vi "Ctor.vi"(8 "error in (no error)":errorcluster) -> (0 "error out":errorcluster, 3 "nmea out":refnum<class "nmea.lvclass">)   [LabVIEW 2012, in "nmea.lvlib" / "nmea.lvclass"]
uses:
  nmea.lvclass
  Ref Data.ctl
  <vilib>/Utility/miscctls.llb/LVDateTimeRec.ctl
  Satellite.ctl
  Fix Type.ctl
  DOP.ctl
  Fix Mode.ctl
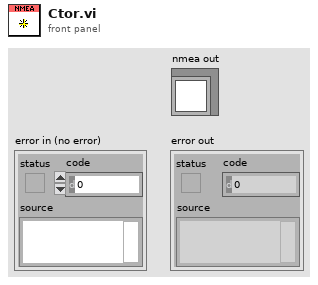
[diagram p1: front panel]
types:
  T1 = typedef "nmea.lvlib/nmea.lvclass/Ref Data.ctl" = cluster{"Latitude":dbl, "Longitude":dbl, "Time":T2, "Status":string, "Speed":dbl, "Course":dbl, "Mag Var":dbl, "Var Dir":string, "Mode":string, "Satellites":T3[], "Next Satellites":T3[], "Active PRNs":i32[], "Fix Type":T4, "DOP":T5, "Fix Mode":T6, "Altitude":dbl, "Geoid":dbl}
  T2 = typedef "LVDateTimeRec.ctl" = cluster{"fractional second":dbl, "second":i32, "minute":i32, "hour":i32, "day of month":i32, "month":i32, "year":i32, "day of week":i32, "day of year":i32, "DST":i32}
  T3 = typedef "nmea.lvlib/nmea.lvclass/Satellite.ctl" = cluster{"PRN":u8, "Channel":u8, "Elevation":u8, "Azimuth":u16, "SNR":u8, "Active":bool}
  T4 = typedef "nmea.lvlib/nmea.lvclass/Fix Type.ctl" = enum16{"N/A", "None", "2D", "3D"}
  T5 = typedef "nmea.lvlib/nmea.lvclass/DOP.ctl" = cluster{"P":dbl, "H":dbl, "V":dbl}
  T6 = typedef "nmea.lvlib/nmea.lvclass/Fix Mode.ctl" = enum16{"Manual", "Auto 2/3D"}
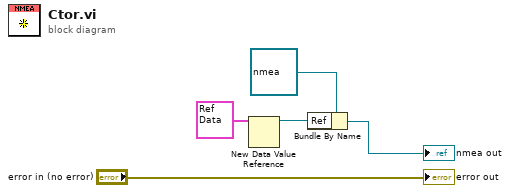
[diagram p0: block diagram]
diagram:
  n1 = New Data Value Reference(data value=T1 {"Latitude"=0.0, "Longitude"=0.0, "Time"={"fractional second"=0.0, "second"=0, "minute"=0, "hour"=0, "day of month"=0, "month"=0, "year"=0, "day of week"=0, "day of year"=0, "DST"=0}, "Status"="", "Speed"=0.0, "Course"=0.0, "Mag Var"=0.0, "Var Dir"="", "Mode"="", "Satellites"=[], "Next Satellites"=[], "Active PRNs"=[], "Fix Type"=enum."N/A", "DOP"={"P"=0.0, "H"=0.0, "V"=0.0}, "Fix Mode"=enum."Manual", "Altitude"=0.0, "Geoid"=0.0} ("Ref Data")) -> (data value reference=w1:refnum<data-value>)  [unwired: 1 in, 1 out]
  n2 = Bundle By Name(cluster=refnum<class "nmea.lvclass"> refnum ("nmea in"), "Ref"=w1) -> (→"nmea out":refnum<class "nmea.lvclass">)
  "error out" <- "error in (no error)"
